vi "Default Group Select.vi"(8 "error in":errorcluster, 11 "Cfg with Chassis":T1) -> (0 "error out":errorcluster, 3 "Selected Grp":T2)   [LabVIEW 2018, in "Configuration Grandmaster.lvlib" / "Cfg Grandmaster.lvclass"]
uses:
  Cfg Grandmaster.lvclass
  Common/Controls/Selected Group.ctl
  Common/Controls/TE_Designator.ctl
  Custom Ctrls/Master Cfg/ge_Cfg wChassis.ctl
  Class Chassis Cfg/ChassisCfg.lvclass
  Class Chassis BOM/Chassis BOM.lvclass
  Data Acquisition/Class Chassis Tasks/Chassis Tasks.lvclass
  Class Timing Group/TimingGrp.lvclass
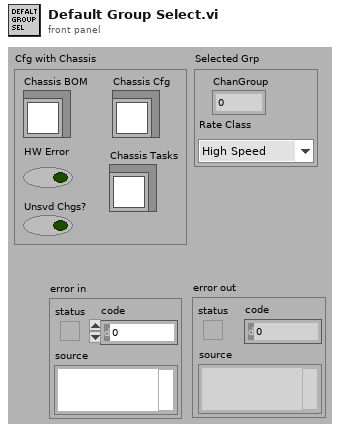
[diagram p1: front panel]
types:
  T1 = typedef "ge_Cfg wChassis.ctl" = cluster{"Chassis BOM":refnum<class "Chassis BOM.lvclass">, "Chassis Cfg":refnum<class "ChassisCfg.lvclass">, "Chassis Tasks":refnum<class "Chassis Tasks.lvclass">, "HW Error":bool, "Unsvd Chgs?":bool}
  T2 = typedef "Selected Group.ctl" = cluster{"ChanGroup":i32, "Rate Class":T3}
  T3 = typedef "TE_Designator.ctl" = enum16{"High Speed", "Low Speed"}
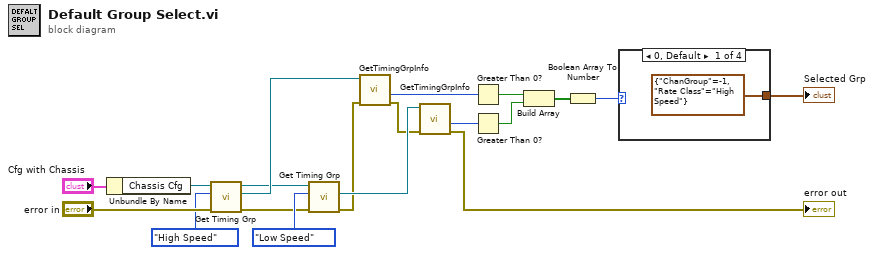
[diagram p0: block diagram]
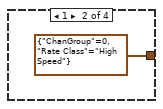
[diagram p2: hidden frame]
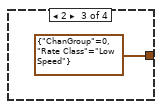
[diagram p3: hidden frame]
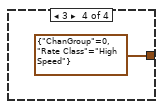
[diagram p4: hidden frame]
diagram:
  n1 = Unbundle By Name("Cfg with Chassis") -> ("Chassis Cfg"=w1:refnum<class "ChassisCfg.lvclass">)
  n2 = call "Get Timing Grp.vi"("error in (no error)"="error in", "Timing Engine"=TE_Designator."High Speed", "Chassis Cfg"=w1) -> ("error out"=w4:errorcluster, "Timing Groups"=w9:refnum<class "TimingGrp.lvclass">, "Chassis Cfg"=w5:refnum<class "ChassisCfg.lvclass">)  [unwired: 6 in]
  n3 = call "Get Timing Grp.vi"("error in (no error)"=w4, "Timing Engine"=TE_Designator."Low Speed", "Chassis Cfg"=w5) -> ("error out"=w3:errorcluster, "Timing Groups"=w7:refnum<class "TimingGrp.lvclass">)  [unwired: 6 in, 1 out]
  n4 = call "GetTimingGrpInfo.vi"("error in"=w3, "TimingGrp in"=w9) -> ("error out"=w2:errorcluster, "Num of Chans"=w14:i32)  [unwired: 4 in, 4 out]
  n5 = call "GetTimingGrpInfo.vi"("error in"=w2, "TimingGrp in"=w7) -> ("error out"=→"error out":errorcluster, "Num of Chans"=w13:i32)  [unwired: 4 in, 4 out]
  n6 = Greater Than 0?(x=w14) -> (x > 0?=w15:bool)
  n7 = Greater Than 0?(x=w13) -> (x > 0?=w16:bool)
  n8 = Build Array(w15, w16) -> (w17:bool[])
  n9 = Boolean Array To Number(Boolean array=w17) -> (number=w18:u32)
  n10 = case shown="0, Default" w18 {
    tunnel: [T2 {"ChanGroup"=-1, "Rate Class"=enum."High Speed"} ("Selected Grp") T2 {"ChanGroup"=0, "Rate Class"=enum."High Speed"} ("Selected Grp") T2 {"ChanGroup"=0, "Rate Class"=enum."Low Speed"} ("Selected Grp") T2 {"ChanGroup"=0, "Rate Class"=enum."High Speed"} ("Selected Grp")] -> w19
    frame 0, Default {
    }
    frame 1 {
    }
    frame 2 {
    }
    frame 3 {
    }
  }
  "Selected Grp" <- w19
